vi "Get Size of Data from TD - Variant (Boxed Empty) - Returns Correct Size.vi"() -> ()   [LabVIEW 2017, in "Composition.Tests.lvlib"]
uses:
  Composition.Tests.lvlib
  <vilib>/addons/_JKI Toolkits/Caraya/classes/Assert/Assert Equal Value_Variant.vi
  Composition/Composition.lvlib
  <vilib>/addons/_JKI Toolkits/Caraya/classes/Test/Test.lvclass
  <vilib>/addons/_JKI Toolkits/Caraya/classes/Assert/Assert.lvclass
panel:
  out "error out":errorcluster
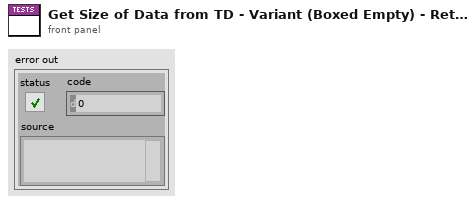
[diagram p1: front panel]
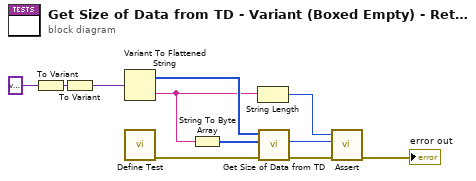
[diagram p0: block diagram]
diagram:
  n1 = To Variant(anything=variant) -> (Variant=w2:variant)
  n2 = To Variant(anything=w2) -> (Variant=w10:variant)
  n3 = Variant To Flattened String(Variant=w10) -> (data string=w3:string, 1:w4:i16[])
  n4 = call <vilib>:"Define Test.vi"() -> ("error out"=w9:errorcluster)  [unwired: 10 in, 1 out]
  n5 = String To Byte Array(string=w3) -> (unsigned byte array=w11:u8[])
  n6 = String Length(string=w3) -> (length=w5:i32)
  n7 = call "Get Size of Data from TD.vi"("error in (no error)"=w9, "Data String"=w11, "Type Descriptor"=w4) -> ("error out"=w8:errorcluster, "Size of Data"=w7:i32)  [unwired: 7 in]
  n8 = call-poly <vilib>:"Assert.vi"("error in (no error)"=w8, "Y"=w7, "X"=w5) -> ("error out"=→"error out":errorcluster)  [unwired: 7 in, 1 out]
